vi "Reset.vi"(8 "error in (no error)":errorcluster, 11 "TesteractHAL_DigitalOutput_NIDAQmx In":refnum<class "TesteractHAL_DigitalOutput_NIDAQmx.lvclass">) -> (0 "error out":errorcluster, 3 "TesteractHAL_DigitalOutput_NIDAQmx Out":refnum<class "TesteractHAL_DigitalOutput_NIDAQmx.lvclass">)   [LabVIEW 2017, in "TesteractHAL_DigitalOutput_NIDAQmx.lvlib" / "TesteractHAL_DigitalOutput_NIDAQmx.lvclass"]
uses:
  TesteractHAL_DigitalOutput_NIDAQmx.lvclass
  TesteractHAL_DigitalOutput_NIDAQmx.lvclass/TesteractHAL_DigitalOutput_NIDAQmx.ctl
  <resource>/objmgr/daqmx.rc
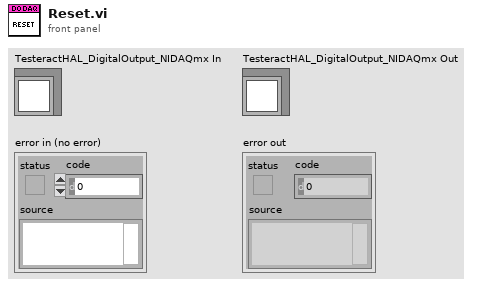
[diagram p1: front panel]
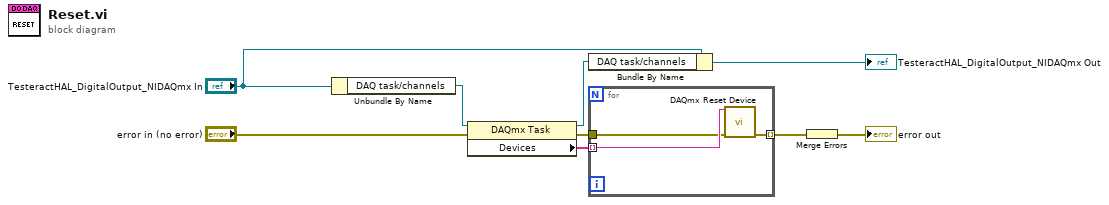
[diagram p0: block diagram]
diagram:
  n1 = Unbundle By Name("TesteractHAL_DigitalOutput_NIDAQmx In") -> ("DAQ task/channels"=w5:refnum<k21>)
  n2 = property class="DAQmx Task"(reference=w5, error in="error in (no error)") -> (reference out=w1:refnum<k21>, error out=w7:errorcluster, "Devices"=w8:tag[])
  n3 = Bundle By Name(cluster="TesteractHAL_DigitalOutput_NIDAQmx In", "DAQ task/channels"=w1) -> (→"TesteractHAL_DigitalOutput_NIDAQmx Out":refnum<class "TesteractHAL_DigitalOutput_NIDAQmx.lvclass">)
  n4 = for {
    tunnel: w8 -> [w11] mode=indexing
    tunnel: w7 -> [w10]
    tunnel: [w12] -> w9 mode=indexing
    n5 = call <vilib>:"DAQmx Reset Device.vi"("device in"=w11, "error in"=w10) -> ("error out"=w12:errorcluster)  [unwired: 13 in]
  }
  n6 = Merge Errors(w9) -> (→"error out":errorcluster)
